vi "niRFUtil CONV 1 Ohm Voltage to 1 Ohm Watt (complex scalar).vi"(7 "Complex Scalar (V)":csg format="%.2f") -> (8 "Real Scalar (W)":sgl format="%.2f")   [LabVIEW 2015, in "niRFUtil.lvlib"]
doc: "(c) Copyright 2006, National Instruments, Inc. This VI may not be duplicated, sold, or distributed without written consent from National Instruments."
uses:
  niRFUtil.lvlib
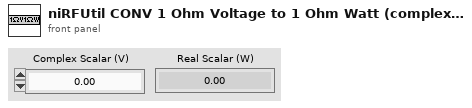
[diagram p1: front panel]
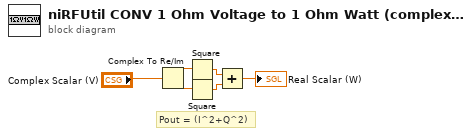
[diagram p0: block diagram]
diagram:
  # "Pout = (I^2+Q^2)"
  n1 = Complex To Re/Im(x + iy="Complex Scalar (V)") -> (x=w6:sgl, y=w5:sgl)
  n2 = Square(x=w6) -> (x^2=w4:sgl)
  n3 = Square(x=w5) -> (x^2=w3:sgl)
  n4 = Add(x=w4, y=w3) -> (x+y=→"Real Scalar (W)":sgl)
